vi "niTuner Get Cal.vi"   [LabVIEW 2011]
doc: "This polymorphic VI returns calibration information for each frequency entry in the scan list. Each frequency entry returns an RF calibration coefficient, an IF calibration coefficient, and (if include attenuation is set to TRUE) a total attenuation calibration coefficient. If there is only a single scan list entry, you can use the Get Cal (single) version of this VI, but if there is more than one scan list entry you must use the Get Cal (multi) version. To select the Get Cal (multi) version, right-click on the icon in your diagram and click <B>select type»Get Cal (multi).vi.</B>"
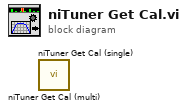
[diagram p0: block diagram]
diagram:
  n1 = call <instrlib>:"niTuner Get Cal (multi).vi"() -> ()  [unwired: 9 in, 3 out]
  n2 = call <instrlib>:"niTuner Get Cal (single).vi"() -> ()  [unwired: 9 in, 3 out]
